vi "Legendre Polynomial_Smm (1D).vi"(8 "m":i32, 11 "X In":dbl[](array[numeric])) -> (0 "2m+1":dbl, 2 "X Out":dbl[](array[numeric]), 3 "Smm(X)":dbl[](array[numeric]))   [LabVIEW 2017, in "NI_AAL_Polynomial.lvlib"]
uses:
  <vilib>/Analysis/NI_AAL_Polynomial.lvlib
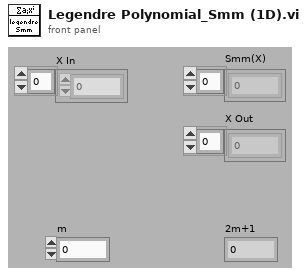
[diagram p1: front panel]
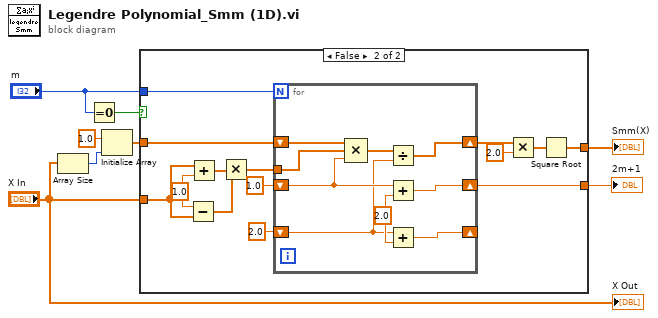
[diagram p0: block diagram]
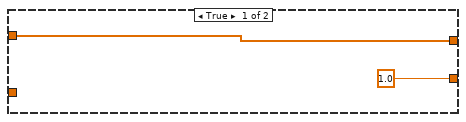
[diagram p2: hidden frame]
diagram:
  n1 = Array Size(array="X In") -> (size(s)=w2:i32)
  n2 = Equal To 0?(x="m") -> (x = 0?=w7:bool)
  n3 = Initialize Array(1.0 ("element"), w2) -> (w4:dbl[])
  n4 = case shown="False" w7 {
    tunnel: "X In" -> [_ w24]
    tunnel: "m" -> [_ w19]
    tunnel: [w10 w11] -> w5
    tunnel: [1.0 ("element") w18] -> w6
    tunnel: w4 -> [w10 w17]
    frame True {
    }
    frame False {
      w23 = 1.0
      n5 = Subtract(x=w23, y=w24) -> (x-y=w21:dbl[])
      n6 = Add(x=w24, y=w23) -> (x+y=w22:dbl[])
      n7 = Multiply(x=w22, y=w21) -> (x*y=w14:dbl[])
      n8 = for {
        N: w19 -> [_]
        shift-right: [w30] -> w18
        shift-left: 1.0 ("element") -> [w31]
        shift-right: [w26] -> w16
        shift-left: w17 -> [w33]
        tunnel: w14 -> [w32]
        shift-right: [w29] -> _
        shift-left: 2.0 ("element") -> [w25]
        w28 = 2.0 ("y")
        n9 = Compound Arithmetic op=MULTIPLY(w33, w32, w31) -> (w27:dbl[])
        n10 = Divide(x=w27, y=w25) -> (x/y=w26:dbl[])
        n11 = Add(x=w31, y=w28) -> (x+y=w30:dbl)
        n12 = Add(x=w25, y=w28) -> (x+y=w29:dbl)
      }
      n13 = Multiply(x=w16, y=2.0) -> (x*y=w13:dbl[])
      n14 = Square Root(x=w13) -> (sqrt(x)=w11:dbl[])
    }
  }
  "2m+1" <- w6
  "Smm(X)" <- w5
  "X Out" <- "X In"
